vi "UI Error Handler - Monitoring.vi"(8 "error in (no error)":errorcluster, 11 "Message Queue":refnum<queue>) -> (3 "dup Message Queue":refnum<queue>)   [LabVIEW 2022 SP3]
uses:
  Message Queue/Message Queue.lvlib
  Message Queue/Message Cluster.ctl
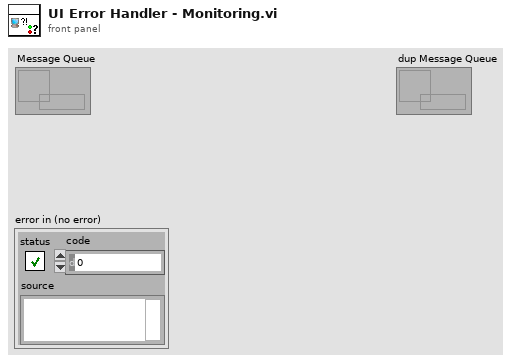
[diagram p1: front panel]
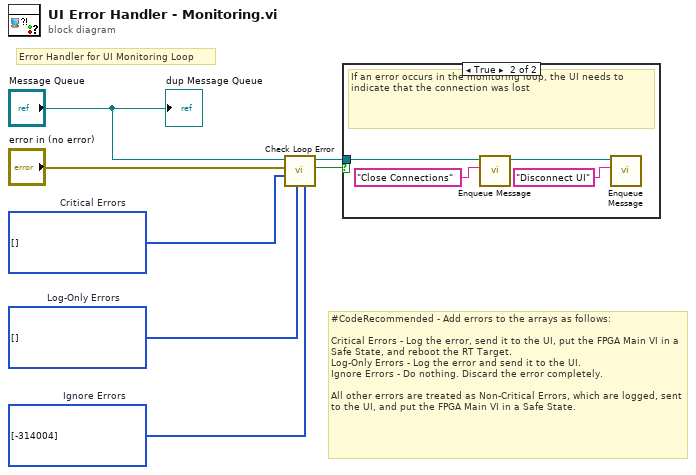
[diagram p0: block diagram]
diagram:
  w5 = i32[] [-314004]  # Ignore Errors
  w6 = i32[] []  # Log-Only Errors
  w7 = i32[] []  # Critical Errors
  # "#CodeRecommended - Add errors to the arrays as follows:\n\nCritical Errors - Log the error, send it to the UI, put the FPGA Main VI in a Safe State, and reboot the RT Target.\nLog-Only Errors - Log the error and send it to the UI.\nIgnore Errors - Do nothing. Discard the error completely.\n\nAll other errors are treated as Non-Critical Errors, which are logged, sent to the UI, and put the FPGA Main VI in a Safe State."
  # "Error Handler for UI Monitoring Loop"
  n1 = call "Check Loop Error.vi"("Ignore Errors"=w5, "Log-Only Errors"=w6, "Critical Errors"=w7, "error to process"="error in (no error)", "Message Queue"="Message Queue") -> ("Enqueued Error?"=w1:bool, "dup Message Queue"=w2:refnum<queue>)  [unwired: 5 in]
  n2 = case shown="True" w1 {
    tunnel: w2 -> [_ w11]
    frame False {
      # "No Error"
    }
    frame True {
      # "If an error occurs in the monitoring loop, the UI needs to indicate that the connection was lost"
      n3 = call "Enqueue Message.vi"("Message"="Close Connections", "Message Queue"=w11) -> ("dup Message Queue"=w9:refnum<queue>)  [unwired: 8 in, 1 out]
      n4 = call "Enqueue Message.vi"("Message"="Disconnect UI", "Message Queue"=w9) -> ()  [unwired: 8 in, 2 out]
    }
  }
  "dup Message Queue" <- "Message Queue"
